vi "pmu_Check Scale Factors CFG-3.vi"(7 "data format":u16, 8 "error in (no error)":errorcluster, 10 "analog channels":T2[](array[typedef]), 11 "phasor channels":T1[](array[typedef]) {"phasor unit" items=["Voltage [V]"=0, "Current [A]"=16777216]; "data modification flag" format="%016b"}) -> (0 "error out":errorcluster)   [LabVIEW 2014, in "NI_EP_PMU.lvlib"]
uses:
  <vilib>/addons/Electrical Power/PMU/NI_EP_PMU.lvlib
  <vilib>/addons/Electrical Power/PMU/Common/Controls/pmu_CFG-3 Analog Channels.ctl
  <vilib>/addons/Electrical Power/PMU/Common/Controls/pmu_CFG-3 Phasor Channels.ctl
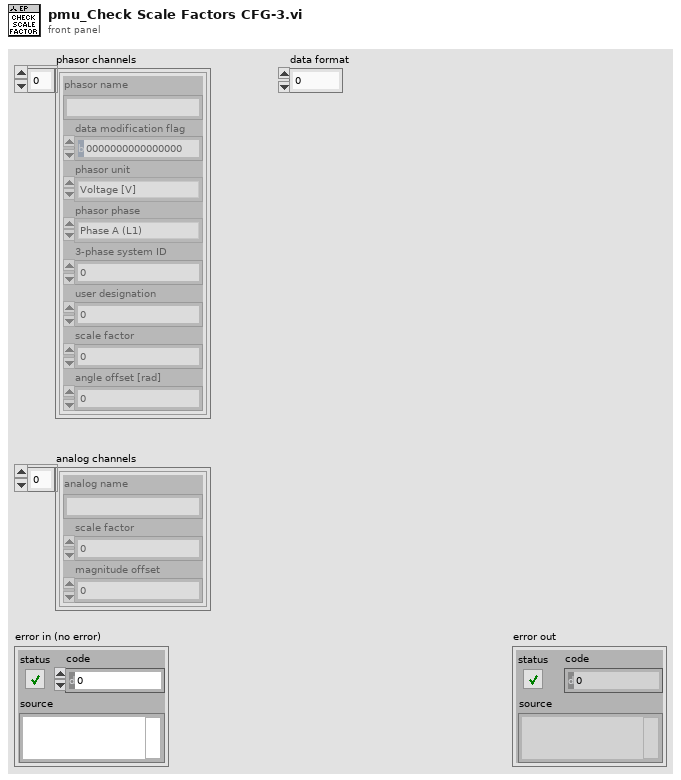
[diagram p1: front panel]
types:
  T1 = typedef "NI_EP_PMU.lvlib/pmu_CFG-3 Phasor Channels.ctl" = cluster{"phasor name":string, "data modification flag":u16, "phasor unit":u32, "phasor phase":enum16{"Phase A (L1)", "Phase B (L2)", "Phase C (L3)", "Phase N", "Positive sequence", "Negative sequence", "Zero sequence"}, "3-phase system ID":u8, "user designation":u8, "scale factor":sgl, "angle offset [rad]":sgl}
  T2 = typedef "NI_EP_PMU.lvlib/pmu_CFG-3 Analog Channels.ctl" = cluster{"analog name":string, "scale factor":sgl, "magnitude offset":sgl}
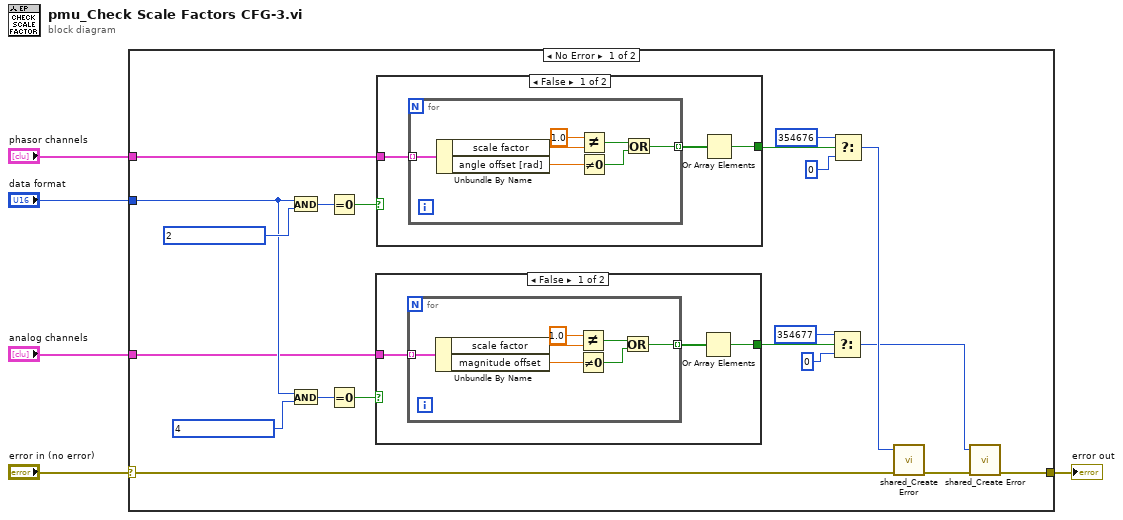
[diagram p0: block diagram]
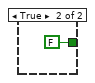
[diagram p2: hidden frame]
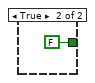
[diagram p3: hidden frame]
diagram:
  n1 = case shown="No Error" "error in (no error)" {
    selector: "error in (no error)" -> [w14 w48]
    tunnel: "phasor channels" -> [w25 _]
    tunnel: "data format" -> [w19 _]
    tunnel: "analog channels" -> [w18 _]
    tunnel: [w8 w48] -> w1
    frame No Error {
      n2 = And(x=w19, y=u16 2 ("x")) -> (x .and. y?=w23:u16)
      n3 = And(x=w19, y=u16 4 ("x")) -> (x .and. y?=w21:u16)
      n4 = Equal To 0?(x=w23) -> (x = 0?=w22:bool)
      n5 = Equal To 0?(x=w21) -> (x = 0?=w17:bool)
      n6 = case shown="False" w17 {
        tunnel: w18 -> [w28 _]
        tunnel: [w26 FALSE] -> w15
        frame False {
          n7 = for {
            tunnel: w28 -> [w35] mode=indexing
            tunnel: [w29] -> w27 mode=indexing
            n8 = Unbundle By Name(w35) -> ("scale factor"=w33:sgl, "magnitude offset"=w34:sgl)
            n9 = Not Equal?(x=sgl 1.0, y=w33) -> (x != y?=w31:bool)
            n10 = Not Equal To 0?(x=w34) -> (x != 0?=w30:bool)
            n11 = Or(x=w31, y=w30) -> (x .or. y?=w29:bool)
          }
          n12 = Or Array Elements(Boolean array=w27) -> (logical OR=w26:bool)
        }
        frame True {
        }
      }
      n13 = case shown="False" w22 {
        tunnel: w25 -> [w39 _]
        tunnel: [w37 FALSE] -> w16
        frame False {
          n14 = for {
            tunnel: w39 -> [w46] mode=indexing
            tunnel: [w40] -> w38 mode=indexing
            n15 = Unbundle By Name(w46) -> ("scale factor"=w44:sgl, "angle offset [rad]"=w45:sgl)
            n16 = Not Equal?(x=sgl 1.0, y=w44) -> (x != y?=w42:bool)
            n17 = Not Equal To 0?(x=w45) -> (x != 0?=w41:bool)
            n18 = Or(x=w42, y=w41) -> (x .or. y?=w40:bool)
          }
          n19 = Or Array Elements(Boolean array=w38) -> (logical OR=w37:bool)
        }
        frame True {
        }
      }
      n20 = Select(t=354677, s=w15, f=0 ("error code (0)")) -> (s? t:f=w9:i32)
      n21 = Select(t=354676, s=w16, f=0 ("error code (0)")) -> (s? t:f=w11:i32)
      n22 = call <vilib>:"shared_Create Error.vi"("error in (no error)"=w14, "error code (0)"=w11) -> ("error out"=w10:errorcluster)  [unwired: 9 in]
      n23 = call <vilib>:"shared_Create Error.vi"("error in (no error)"=w10, "error code (0)"=w9) -> ("error out"=w8:errorcluster)  [unwired: 9 in]
    }
    frame Error {
    }
  }
  "error out" <- w1
